vi "ABR-Set Level.vi"(0 "Runtime":T1, 11 "error in (no error)":errorcluster) -> (4 "Runtime thru":T1, 14 "Level":dbl, 15 "error out":errorcluster)   [LabVIEW 2020]
uses:
  Typedefs/ABR-Runtime Data.ctl
  epl-vi-lib/Signal Synthesis VIs/4th Generation/Classes/SignalManager/SignalManager.lvclass
  epl-vi-lib/PXI DAQ VIs/AODO/Typedefs/AODO-Action.ctl
  epl-vi-lib/Signal Synthesis VIs/4th Generation/Classes/SignalManager/SignalManager.lvclass/SignalManager.ctl
  epl-vi-lib/Signal Synthesis VIs/4th Generation/Classes/SignalManager/Read Channels.vi
  epl-vi-lib/Signal Synthesis VIs/4th Generation/Classes/Channel/Channel.lvclass
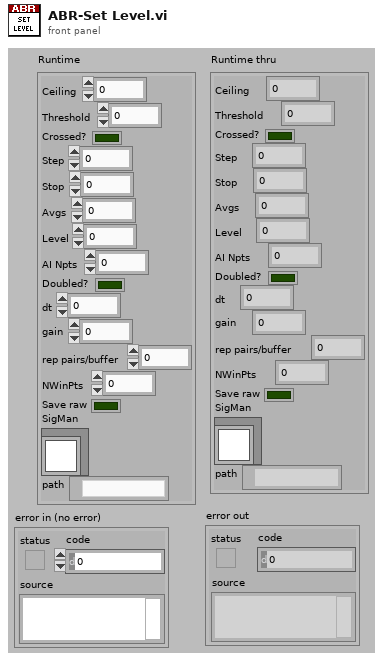
[diagram p1: front panel]
types:
  T1 = typedef "ABR-Runtime Data.ctl" = cluster{"Ceiling":dbl, "Threshold":dbl, "Crossed?":bool, "Step":dbl, "Stop":i32, "Avgs":i32, "Level":dbl, "AI Npts":i32, "Doubled?":bool, "dt":dbl, "gain":dbl, "rep pairs/buffer":i32, "NWinPts":i32, "Save raw":bool, "SigMan":refnum<class "SignalManager.lvclass">, "path":path}
  T2 = typedef "AODO-Action.ctl" = enum16{"Configure", "Initialize", "Start", "Write", "Clean up", "Init & Start", "Config & Test", "Position", "Set AO Gains", "Zero", "Prime", "Status"}
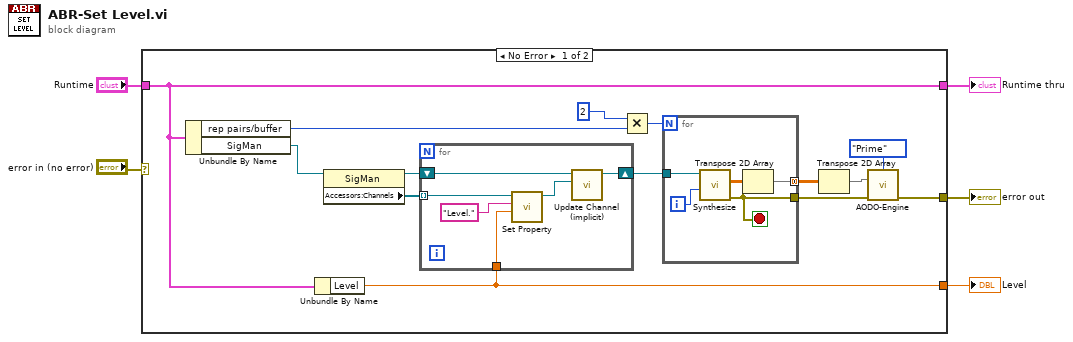
[diagram p0: block diagram]
diagram:
  n1 = case shown="No Error" "error in (no error)" {
    selector: "error in (no error)" -> [_ w31]
    tunnel: "Runtime" -> [w10 w32]
    tunnel: [w10 w32] -> w3
    tunnel: [w16 w31] -> w2
    tunnel: [w9 _] -> w1
    frame No Error {
      n2 = Unbundle By Name(w10) -> ("rep pairs/buffer"=w13:i32, "SigMan"=w7:refnum<class "SignalManager.lvclass">)
      n3 = Unbundle By Name(w10) -> ("Level"=w9:dbl)
      n4 = property class="SigMan"(reference=w7) -> (reference out=w12:refnum<class "SignalManager.lvclass">, "Accessors:Channels"=w11:refnum<class "Channel.lvclass">[])  [unwired: 1 in, 1 out]
      n5 = for {
        tunnel: w11 -> [w23] mode=indexing
        shift-right: [w24] -> w8
        shift-left: w12 -> [w25]
        tunnel: w9 -> [w21]
        n6 = call "Set Property.vi"("Value"=w21, "Property"="Level.", "Channel in"=w23) -> ("Channel out"=w20:refnum<class "Channel.lvclass">)  [unwired: 7 in, 1 out]
        n7 = call "Update Channel (implicit).vi"("Channel"=w20, "SignalManager in"=w25) -> ("SignalManager out"=w24:refnum<class "SignalManager.lvclass">)  [unwired: 8 in, 1 out]
      }
      n8 = Multiply(x=2 ("y"), y=w13) -> (x*y=w18:i32)
      n9 = for {
        N: w18 -> [_]
        tunnel: w8 -> [w30]
        tunnel: [w26] -> w15 mode=concatenating
        tunnel: [w27] -> w17
        i -> [w29]
        stop <- w27 stop-if-true
        n10 = call "Synthesize.vi"("Repetition"=w29, "SigMan in"=w30) -> ("error out"=w27:errorcluster, "Array"=w28:dbl[][])  [unwired: 7 in, 1 out]
        n11 = Transpose 2D Array(2D array=w28) -> (transposed array=w26:dbl[][])
      }
      n12 = Transpose 2D Array(2D array=w15) -> (transposed array=w6:dbl[][])
      n13 = call "AODO-Engine.vi"("Action"=AODO-Action."Prime", "AO"=w6, "error in (no error)"=w17) -> ("error out"=w16:errorcluster)  [unwired: 7 in, 5 out]
    }
    frame Error {
    }
  }
  "error out" <- w2
  "Level" <- w1
  "Runtime thru" <- w3
